vi "interop.vi"() -> ()   [LabVIEW 2022 SP3]
uses:
  return value.ctl
  <vilib>/Utility/error.llb/DialogType.ctl
  cluster.ctl
  cluster 2.ctl
panel:
  out "return array":T1[](array[typedef])
  out "return value":T1
  in  "Python version":string="3.9"
  out "String":string
  in  "module path":path=path "C:/Users/Mikio Fukushima/Desktop/work/Kabushima/LabVIEW-and-Python-interop/interop/interop.py"
  in  "error in":errorcluster
  out "error out":errorcluster
  in  "Python path":path=path "C:/Users/Mikio Fukushima/AppData/Local/Programs/Python/Python39/python.exe"
  # "pythonスクリプトのパスに2バイトコードを含めるとエラーになるので注意。"
  # "LabVIEW.iniに\nShowConsoleForPythonNode=TRUE\nを追加すると、Pythonノード実行時にコンソールが開いて標準出力を見る事が出来る。"
  # "Pythonノードを使用したLabVIEWへの/LabVIEWからのPythonデータ構造の受け渡し\nhttps://knowledge.ni.com/KnowledgeArticleDetails?id=kA03q000000oyaHCAQ&l=ja-JP"
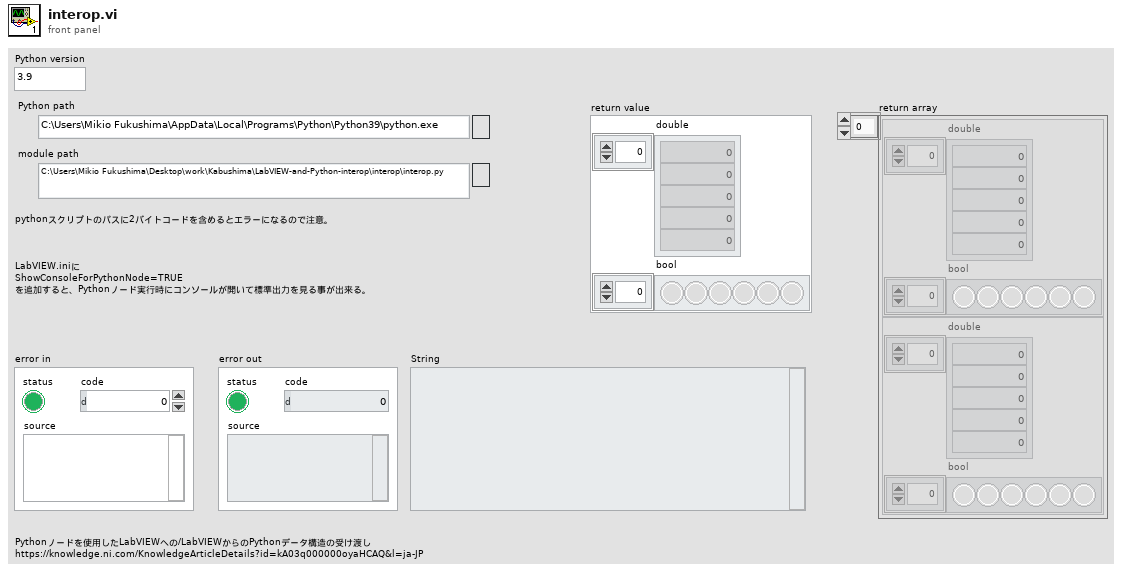
[diagram p1: front panel]
types:
  T1 = typedef "return value.ctl" = cluster{"double":dbl[], "bool":bool[]}
  T2 = typedef "cluster 2.ctl" = cluster{"Enum":enum16{"Item1", "Item2"}}
  T3 = typedef "cluster.ctl" = cluster{"double":dbl, "i32 array":i32[], "String":string, "Cluster 2":T2}
  T4 = typedef "DialogType.ctl" = u16
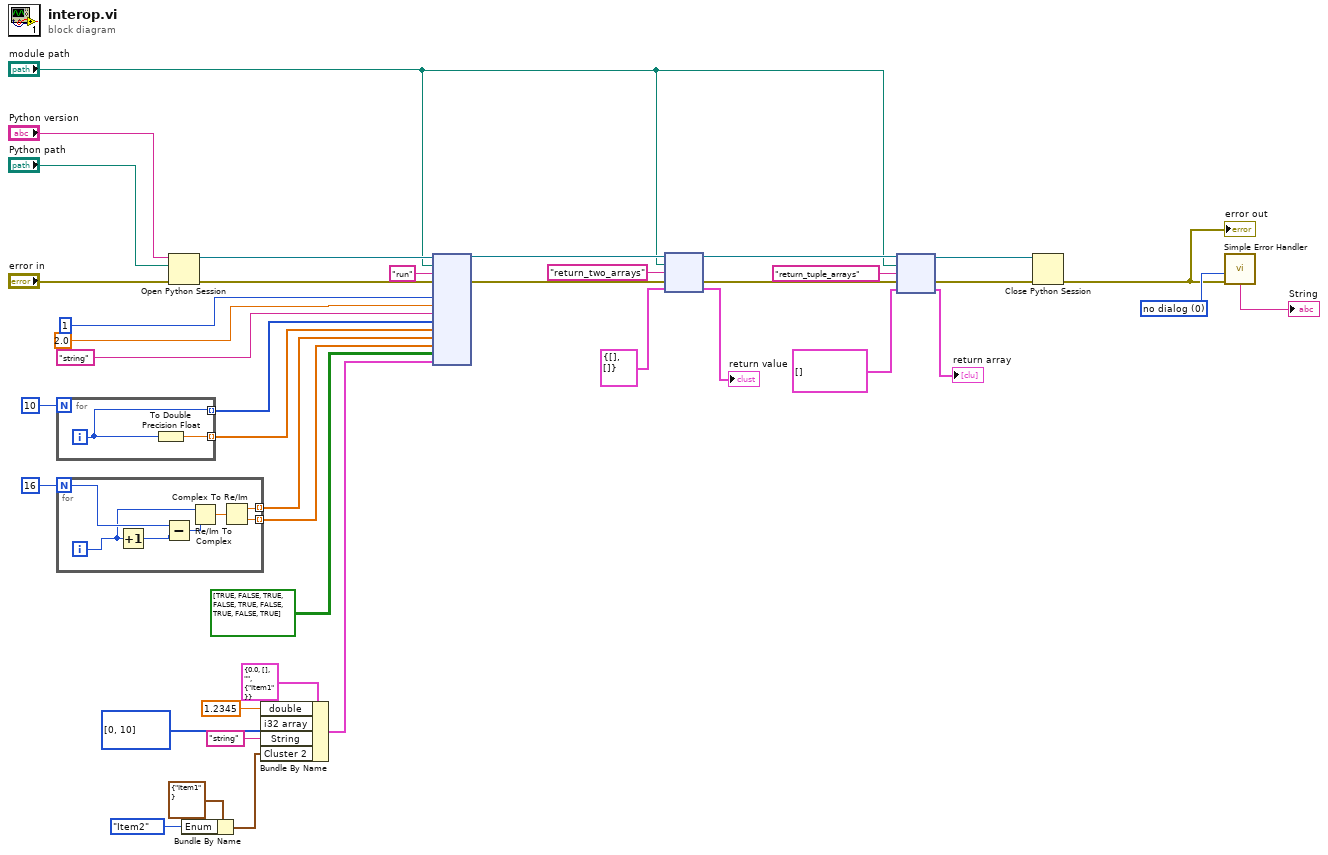
[diagram p0: block diagram]
diagram:
  w36 = T4 0 items=["no dialog", "OK message", "continue or stop message", "OK message + warnings", "continue/stop + warnings"] ("type of dialog (OK msg:1)")
  n1 = for {
    N: 10 -> [_]
    tunnel: [w42] -> w29 mode=indexing
    tunnel: [w41] -> w30 mode=indexing
    i -> [w42]
    n2 = To Double Precision Float(number=w42) -> (double precision float=w41:dbl)
  }
  n3 = for {
    N: 16 -> [w46]
    tunnel: [w49] -> w27 mode=indexing
    tunnel: [w48] -> w28 mode=indexing
    i -> [w45]
    n4 = Increment(x=w45) -> (x+1=w43:i32)
    n5 = Subtract(x=w46, y=w43) -> (x-y=w44:i32)
    n6 = Re/Im To Complex(1:w44, 2:w45) -> (0:w47:cdb)
    n7 = Complex To Re/Im(x + iy=w47) -> (x=w49:dbl, y=w48:dbl)
  }
  n8 = Open Python Session(python version="Python version", python path="Python path", 3:"error in") -> (session out=w39:refnum<k35>, error out=w38:errorcluster)
  n9 = Bundle By Name(cluster=T2 {"Enum"=enum."Item1"} ("Cluster 2"), "Enum"=enum16{"Item1", "Item2"}."Item2") -> (w18:T2)
  n10 = Bundle By Name(cluster=T3 {"double"=0.0, "i32 array"=[], "String"="", "Cluster 2"={"Enum"=enum."Item1"}} ("Cluster"), "double"=1.2345, "i32 array"=i32[] [0, 10], "String"="string", "Cluster 2"=w18) -> (w24:T3)
  n11 = node(w39, "module path", "run" ("function name"), w38, 1, 2.0, "string", w29, w30, w27, w28, bool[][] [[TRUE, FALSE, TRUE], [FALSE, TRUE, FALSE], [TRUE, FALSE, TRUE]], w24) -> (w14:refnum<k35>, w15:errorcluster)  [unwired: 11 in, 2 out]
  n12 = node(w14, "module path", "return_two_arrays" ("function name"), w15, T1 {"double"=[], "bool"=[]} ("return value")) -> (w8:refnum<k35>, w5:errorcluster, →"return value":T1)  [unwired: 2 out]
  n13 = node(w8, "module path", "return_tuple_arrays" ("function name"), w5, T1[] []) -> (w7:refnum<k35>, w6:errorcluster, →"return array":T1[])  [unwired: 2 out]
  n14 = Close Python Session(session in=w7, error in=w6) -> (11:w9:errorcluster)
  "error out" <- w9
  n15 = call <vilib>:"Simple Error Handler.vi"("type of dialog (OK msg:1)"=w36, "error in (no error)"=w9) -> ("message"=→"String":string)  [unwired: 3 in, 4 out]
